vi "SimConfigGlobal.vi"() -> ()   [LabVIEW 2017, in "IrAcquisition.lvlib"]
uses:
  <vilib>/addons/InsightCM/Devices/Shared/Ir/IrAcquisition/IrAcquisition.lvlib
  <vilib>/addons/InsightCM/Devices/Shared/Ir/IrAcquisition/controls/simScaleConfig.ctl
panel:
  in  "Cam2DataName":refnum<vi>
  in  "Cam2ConfigRef":refnum<vi>
  in  "Cam2Ref":refnum<vi>
  in  "Cam2Data":sgl[][](array[numeric])
  in  "Cam2DataSet":string
  in  "Cam1DataName":refnum<vi>
  in  "Cam1ConfigRef":refnum<vi>
  in  "Cam1Ref":refnum<vi>
  in  "Cam1Data":sgl[][](array[numeric])
  in  "Cam1DataSet":string
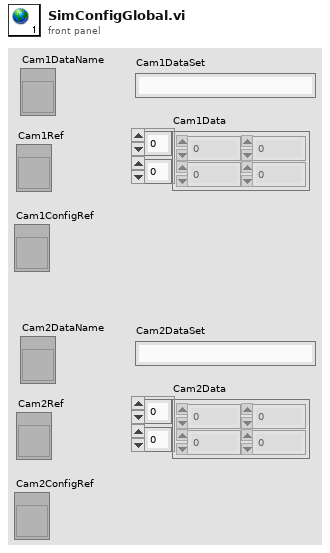
[diagram p1: front panel]
diagram:
